vi "Substitute Message.vi"(10 "Substitute Message":refnum<class "MSG.lvclass">, 11 "Send IN":refnum<class "Send.lvclass">) -> (3 "Observer":refnum<class "Observer.lvclass">)   [LabVIEW 2011, in "Messenging.lvlib" / "Observer.lvclass"]
uses:
  SendOnly/Observer.lvclass
  Send/Send.lvclass
  TextVarientMessage/MSG.lvclass
  Message Translation/Translator/Translator.lvclass
  Message Translation/SubstututeMessage Folder/SubstututeMessage.lvclass
  ObserverSet.lvclass
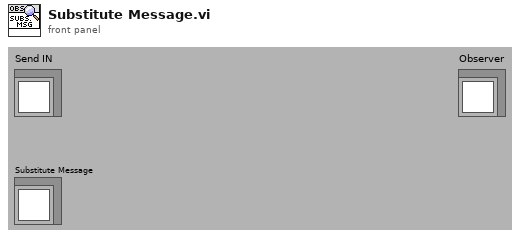
[diagram p1: front panel]
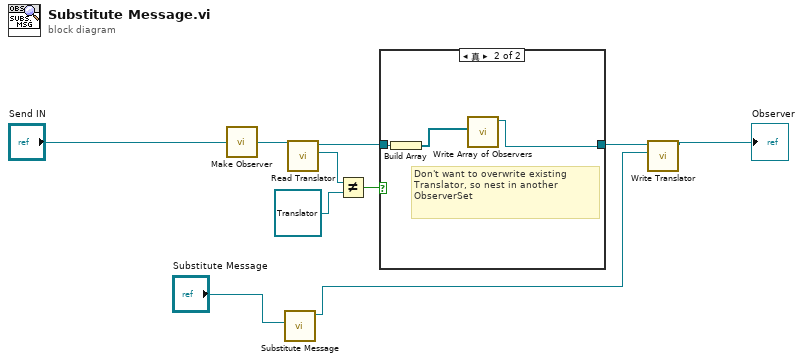
[diagram p0: block diagram]
diagram:
  n1 = call "Make Observer.vi"("To be an Observer"="Send IN") -> ("Observer"=w9:refnum<class "Observer.lvclass">)
  n2 = call "Substitute Message.vi"("Message to Substitute"="Substitute Message") -> ("Translator"=w1:refnum<class "SubstututeMessage.lvclass">)  [unwired: 10 out]
  n3 = call "Read Translator.vi"("Observer.lvclass in"=w9) -> ("Messenging.lvlib:Translator.lvclass"=w7:refnum<class "Translator.lvclass">, "Observer.lvclass out"=w4:refnum<class "Observer.lvclass">)  [unwired: 1 in, 8 out]
  n4 = Not Equal?(x=w7, y=refnum<class "Translator.lvclass"> refnum ("Messenging.lvlib:Translator.lvclass")) -> (x != y?=w6:bool)
  n5 = case shown="真" w6 {
    tunnel: [w11 w12] -> w5
    tunnel: w4 -> [w11 w14]
    frame False {
    }
    frame True {
      # "Don't want to overwrite existing\nTranslator, so nest in another\nObserverSet"
      n6 = Build Array(w14) -> (w13:refnum<class "Observer.lvclass">[])
      n7 = call "Write Array of Observers.vi"("Array of Observers"=w13) -> ("ObserverSet.lvclass out"=w12:refnum<class "ObserverSet.lvclass">)  [unwired: 2 in, 8 out]
    }
  }
  n8 = call "Write Translator.vi"("Messenging.lvlib:Translator.lvclass"=w1, "Observer.lvclass in"=w5) -> ("Observer.lvclass out"=→"Observer":refnum<class "Observer.lvclass">)  [unwired: 1 in, 8 out]
